vi "Read Settings.vi"(8 "error in (no error)":errorcluster, 10 "Settings ID":string, 11 "Configuration Session in":refnum<class "Configuration Session.lvclass">) -> (0 "error out":errorcluster, 1 "value":T1, 3 "Configuration Session out":refnum<class "Configuration Session.lvclass">, 4 "found?":bool)   [LabVIEW 2017, in "DSF Core.lvlib" / "Configuration Session.lvclass"]
doc: "Reads a value associated with a key in a specified section from the configuration data identified by <B>dsf refnum</B>. If the key does not exist, the VI returns the default value. This VI supports multibyte characters in strings. Wire data to the <B>default value</B> input to determine the polymorphic instance to use or manually select the instance."
uses:
  Configuration Session.lvclass
  Typedefs/DSF Settings Info.ctl
  DSF Core.lvlib
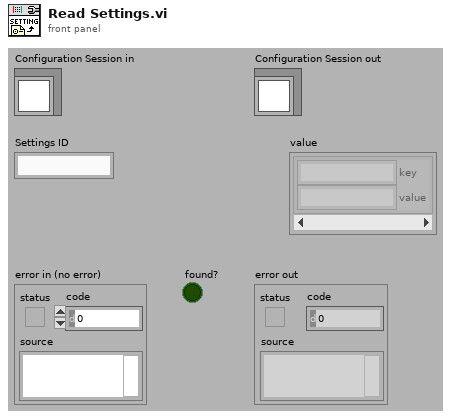
[diagram p1: front panel]
types:
  T1 = typedef "DSF Core.lvlib/DSF Settings Info.ctl" = cluster{"key":string, "value":string}[]
  T2 = typedef "DSF Core.lvlib/Configuration Session.lvclass/DSF Config Data Ref.ctl" = refnum<data-value>
  T3 = typedef "DSF Core.lvlib/Configuration Session.lvclass/DSF Config Data.ctl" = cluster{"path":path, "dirty":bool, "dsf configuration":T4}
  T4 = typedef "DSF Core.lvlib/Configuration Session.lvclass/Internal DSF Configuration.ctl" = cluster{"dsfversion":T5, "version":T5, "framework configuration":T6}
  T5 = typedef "DSF Core.lvlib/DSF Version Info.ctl" = cluster{"major":u32, "minor":u32, "fix":u32, "build":string}
  T6 = typedef "DSF Core.lvlib/Configuration Session.lvclass/DSF Engine Framework JSON Configuration.ctl" = cluster{"Plugins":T7[]}
  T7 = typedef "DSF Core.lvlib/Configuration Session.lvclass/DSF Engine Plugin JSON Configuration.ctl" = cluster{"name":string, "components":string[], "cycle timing":T8, "threads":T9[], "Transfer Groups":T10[], "settings":T1}
  T8 = typedef "DSF Core.lvlib/DSF Timing Info.ctl" = cluster{"priority":u64, "decimation":u64, "offset":u64}
  T9 = typedef "DSF Core.lvlib/DSF Engine Plugin Thread Configuration.ctl" = cluster{"buffer converter settings":T1, "transceiver settings":T1, "custom settings":T1, "processor":i32, "priority offset":i16}
  T10 = typedef "DSF Core.lvlib/Configuration Session.lvclass/DSF Engine Transfer Group JSON Configuration.ctl" = cluster{"name":string, "direction":u8, "cycle timing":T8, "thread index":i32, "settings":T1, "Transfers":T11[], "timeout behavior":u8}
  T11 = typedef "DSF Core.lvlib/Configuration Session.lvclass/DSF Engine Transfer JSON Configuration.ctl" = cluster{"name":string, "byte order":u8, "settings":T1, "channels":T12[]}
  T12 = typedef "DSF Core.lvlib/Configuration Session.lvclass/DSF Engine Channel JSON Configuration.ctl" = cluster{"string offset":u64, "string data type":u8, "engine data type":u8, "name":string, "settings":T1, "units":string}
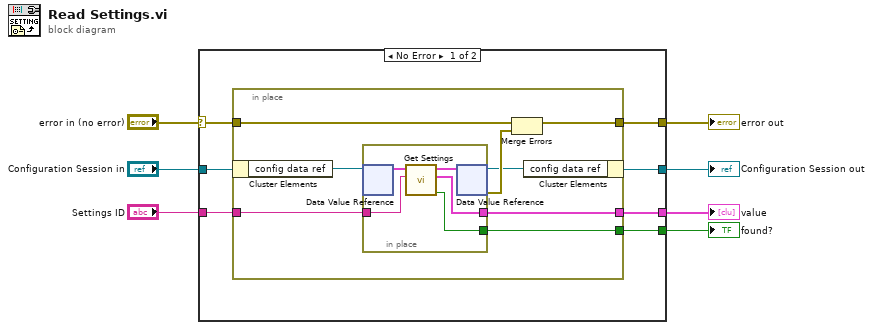
[diagram p0: block diagram]
diagram:
  n1 = case shown="No Error" "error in (no error)" {
    selector: "error in (no error)" -> [w8 w29]
    tunnel: "Settings ID" -> [w14 _]
    tunnel: [w13 _] -> w6
    tunnel: [w12 _] -> w5
    tunnel: "Configuration Session in" -> [w11 w28]
    tunnel: [w10 w29] -> w3
    tunnel: [w9 w28] -> w2
    frame No Error {
      n2 = in-place {
        in-place-border: w14 -> [w22]
        in-place-border: [w21] -> w13
        in-place-border: [w20] -> w12
        in-place-border: w8 -> [w17]
        in-place-border: [w16] -> w10
        n3 = in-place-cluster #1(w11) -> ("config data ref"=w19:T2)
        n4 = in-place {
          in-place-border: w22 -> [w27]
          in-place-border: [w26] -> w21
          in-place-border: [w25] -> w20
          n5 = in-place-dvr #2(w19) -> (w24:T3)  [unwired: 1 out]
          n6 = call "Get Settings.vi"("id"=w27, "DSF Configuration in"=w24) -> ("exists?"=w25:bool, "info"=w26:T1, "DSF Configuration out"=w23:T3)  [unwired: 6 in, 1 out]
          n7 = in-place-dvr #2(w23) -> (w15:T2, w18:errorcluster)
        }
        n8 = Merge Errors(w17, w18) -> (w16:errorcluster)
        n9 = in-place-cluster #1("config data ref"=w15) -> (w9:refnum<class "Configuration Session.lvclass">)
      }
    }
    frame Error {
    }
  }
  "error out" <- w3
  "found?" <- w5
  "value" <- w6
  "Configuration Session out" <- w2
